vi "Mode Facade.vi"(0 "Data In":T5, 2 "Display State In":T3, 3 "Container State":T4) -> (6 "Data Out":T5, 7 "Display State Out":T3, 8 "Action":T2)   [LabVIEW 2013, in "VertMode.xctl"]
uses:
  VertMode.xctl
  Mode Data.ctl
  <vilib>/_xctls/Container State.ctl
  Mode State.ctl
  <vilib>/_xctls/Action.ctl
  <vilib>/_xctls/XControlSupport.lvlib
panel:
  in  "Mode":T1
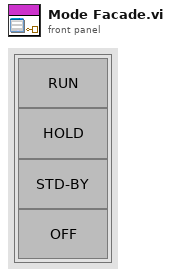
[diagram p1: front panel]
types:
  T1 = cluster{"Off":bool, "Standby":bool, "Hold":bool, "Run":bool}
  T2 = typedef "XControlSupport.lvlib/Action.ctl" = cluster{"Data Changed?":bool, "State Changed?":bool, "Action Name":string}
  T3 = typedef "VertMode.xctl/Mode State.ctl" = cluster{"Numeric":dbl}
  T4 = typedef "XControlSupport.lvlib/Container State.ctl" = cluster{"Indicator?":bool, "Run Mode?":bool, " Refnum":refnum<vi>}
  T5 = typedef "VertMode.xctl/Mode Data.ctl" = enum8{"Off", "Stby", "Hold", "Run"}
  T6 = cluster{"[0]":bool, "[1]":bool, "[2]":bool, "[3]":bool}
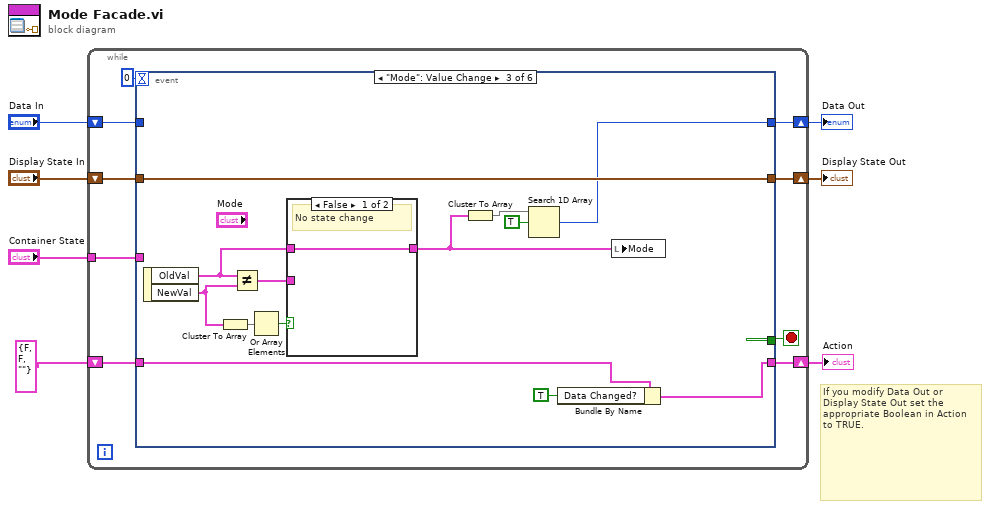
[diagram p0: block diagram]
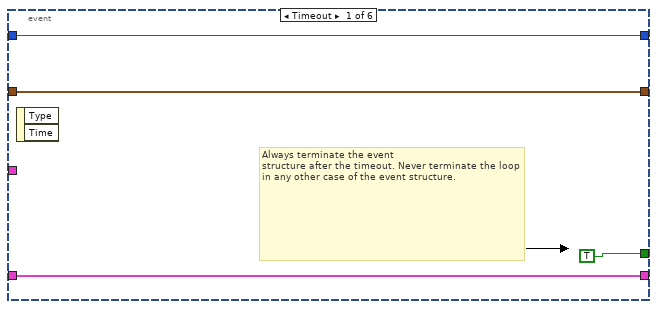
[diagram p2: hidden frame]
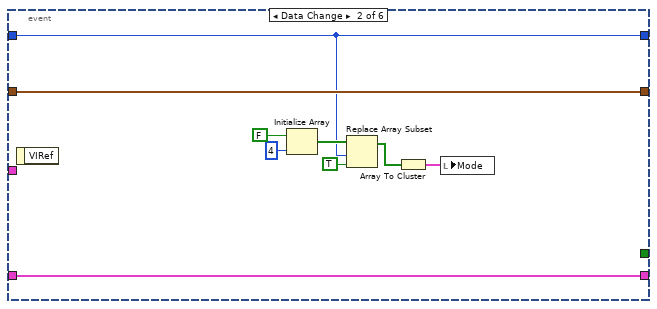
[diagram p3: hidden frame]
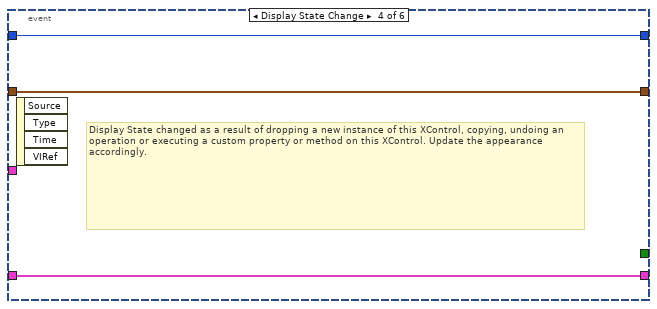
[diagram p5: hidden frame]
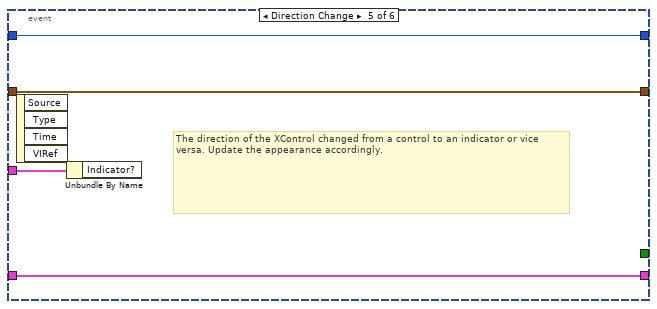
[diagram p6: hidden frame]
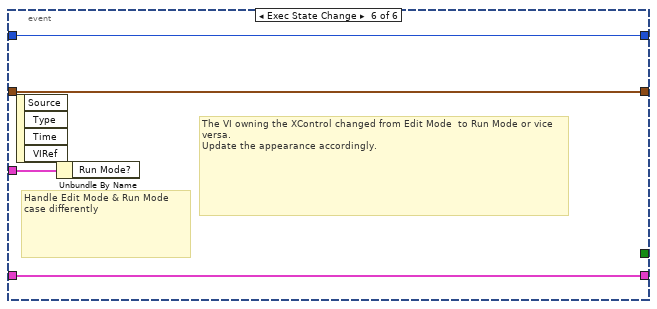
[diagram p7: hidden frame]
diagram:
  # "If you modify Data Out or\nDisplay State Out set the\nappropriate Boolean in Action\nto TRUE."
  n1 = while {
    shift-right: [w15] -> w4
    shift-left: "Display State In" -> [w16]
    tunnel: "Container State" -> [w12]
    shift-right: [w10] -> w7
    shift-left: "Data In" -> [w11]
    shift-right: [w8] -> w2
    shift-left: T2 {"Data Changed?"=FALSE, "State Changed?"=FALSE, "Action Name"=""} ("Action") -> [w9]
    stop <- w14 stop-if-true
    n2 = event shown="[2] \"Mode\": Value Change" {
      selector: _ -> [_ _ _ _ _ _]
      dyn-events: _ -> [_ _ _ _ _ _]
      timeout: 0 -> [_ _ _ _ _ _]
      tunnel: w16 -> [w18 w29 w42 w47 w50 w54]
      tunnel: [w18 w29 w42 w47 w50 w54] -> w15
      tunnel: [TRUE _ _ _ _ _] -> w14
      tunnel: w12 -> [_ _ _ _ w51 w55]
      tunnel: w11 -> [w17 w24 _ w46 w49 w53]
      tunnel: [w17 w24 w33 w46 w49 w53] -> w10
      tunnel: [w19 w28 w30 w45 w48 w52] -> w8
      tunnel: w9 -> [w19 w28 w32 w45 w48 w52]
      event Timeout {
        # "Always terminate the event\nstructure after the timeout. Never terminate the loop in any other case of the event structure."
        n3 = event-data() -> ()  [unwired: 1 in, 2 out]
      }
      event Data Change {
        n4 = event-data() -> ()  [unwired: 1 in, 1 out]
        n5 = Initialize Array(FALSE, 4 ("dimension size")) -> (w25:bool[])
        n6 = Replace Array Subset(array=w25, new element=TRUE ("new element/subarray"), index=w24) -> (w22:bool[])
        n7 = Array To Cluster(array=w22) -> (cluster=w21:T6)
        n8 = local write "Mode"(w21) -> ()
      }
      event "Mode": Value Change {
        n9 = event-data() -> ("OldVal"=w38:T1, "NewVal"=w41:T1)  [unwired: 1 in]
        n10 = Cluster To Array(cluster=w41) -> (array=w40:bool[])
        n11 = Not Equal?(x=w38, y=w41) -> (x != y?=w37:T1)
        n12 = Or Array Elements(Boolean array=w40) -> (logical OR=w39:bool)
        n13 = case shown="False" w39 {
          tunnel: w38 -> [w43 _]
          tunnel: [w43 w44] -> w36
          tunnel: w37 -> [_ w44]
          frame False {
            # "No state change"
          }
          frame True {
          }
        }
        n14 = Cluster To Array(cluster=w36) -> (array=w35:bool[])
        n15 = Search 1D Array(1D array=w35, element=TRUE) -> (index of element=w33:i32)  [unwired: 1 in]
        n16 = Bundle By Name(cluster=w32, "Data Changed?"=TRUE) -> (w30:T2)
        n17 = local write "Mode"(w36) -> ()
      }
      event Display State Change {
        # "Display State changed as a result of dropping a new instance of this XControl, copying, undoing an operation or executing a custom property or method on this XControl. Update the appearance accordingly."
        n18 = event-data() -> ()  [unwired: 1 in, 4 out]
      }
      event Direction Change {
        # "The direction of the XControl changed from a control to an indicator or vice versa. Update the appearance accordingly."
        n19 = event-data() -> ()  [unwired: 1 in, 4 out]
        n20 = Unbundle By Name(w51) -> ()  [unwired: 1 out]
      }
      event Exec State Change {
        # "The VI owning the XControl changed from Edit Mode  to Run Mode or vice versa.\nUpdate the appearance accordingly."
        # "Handle Edit Mode & Run Mode\ncase differently"
        n21 = event-data() -> ()  [unwired: 1 in, 4 out]
        n22 = Unbundle By Name(w55) -> ()  [unwired: 1 out]
      }
    }
  }
  "Display State Out" <- w4
  "Data Out" <- w7
  "Action" <- w2
